vi "lv get dataset by rid.vi"(8 "error in":errorcluster, 10 "dataset rid":string, 11 "client handle":i32) -> (0 "error out":errorcluster, 3 "dataset handle":i32)   [LabVIEW 2026]
uses:
  bin/nominalClient_64.dll
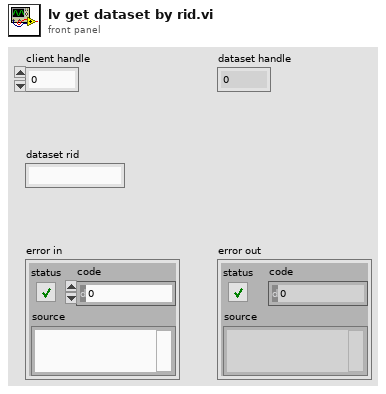
[diagram p1: front panel]
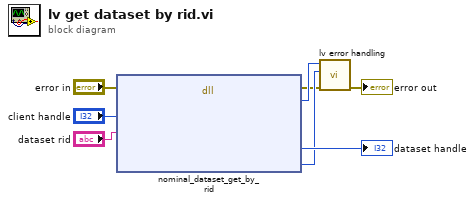
[diagram p0: block diagram]
diagram:
  n1 = dll-call lib="C:/sw/nominal-c/bin/nominalClient_64.dll" fn="nominal_dataset_get_by_rid"(error in="error in", "client"="client handle", "rid"="dataset rid") -> (error out=w1:errorcluster, "return type"=w2:i32, "dataset handle"=→"dataset handle":i32, "errorout"=w3:i32)  [unwired: 6 in, 1 out]
  n2 = call "lv error handling.vi"("error in"=w1, "error handle"=w3, "return code"=w2) -> ("error out"=→"error out":errorcluster)  [unwired: 8 in]
